vi "multiply.vi"(9 "B":dbl, 11 "A":dbl) -> (2 "result":dbl)   [LabVIEW 2020]
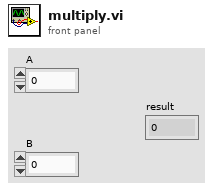
[diagram p1: front panel]
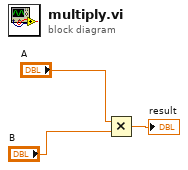
[diagram p0: block diagram]
diagram:
  n1 = Multiply(x="A", y="B") -> (x*y=→"result":dbl)
